vi "_Main.vi"   [LabVIEW 2016, in "System_Status.lvlib"]
uses:
  System_Status.lvlib
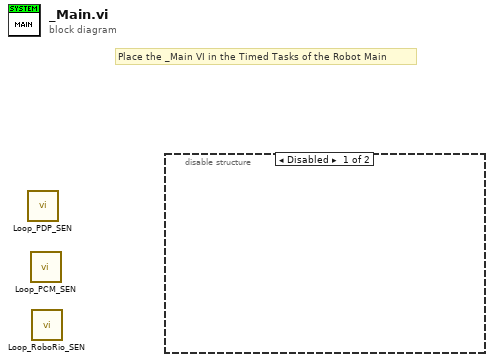
[diagram p0: block diagram]
diagram:
  # "Place the _Main VI in the Timed Tasks of the Robot Main"
  n1 = call "Loop_PDP_SEN.vi"() -> ()  [unwired: 12 in]
  n2 = call "Loop_PCM_SEN.vi"() -> ()  [unwired: 12 in]
  n3 = call "Loop_RoboRio_SEN.vi"() -> ()  [unwired: 12 in]
  n4 = disable-structure shown="Disabled" {
    frame Disabled {
    }
    frame Enabled {
    }
  }
